vi "global.vi"() -> ()   [LabVIEW 2015]
panel:
  out "FG Data":T1
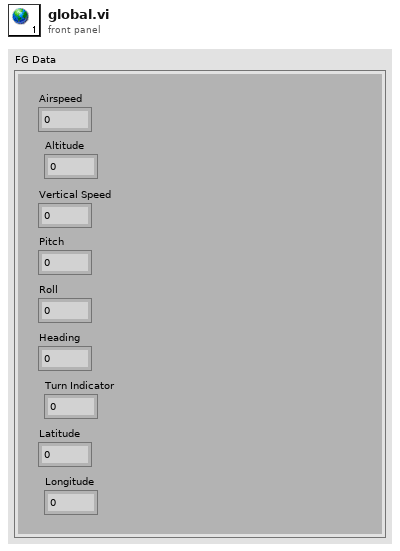
[diagram p1: front panel]
types:
  T1 = cluster{"Airspeed":dbl, "Altitude":dbl, "Vertical Speed":dbl, "Pitch":dbl, "Roll":dbl, "Heading":dbl, "Turn Indicator":dbl, "Latitude":dbl, "Longitude":dbl}
diagram:
